vi "AcquisitionConfig.vi"(0 "frequency settings":T1={"frequency (Hz)"=0.001, "number of samples per cycle"=2.0, "number of cycles"=1.0} {"frequency (Hz)" min=0.001 max=100000000.0; "number of samples per cycle" min=2.0 step=1.0; "number of cycles" min=1.0}, 5 "channel settings":T2={"units"=10348, "input terminal configuration"=-1, "maximum value"=5.0, "minimum value"=-5.0} {"units" items=["Volts"=10348, "From Custom Scale"=10065]; "input terminal configuration" items=["Default"=-1, "RSE"=10083, "NRSE"=10078, "Differential"=10106, "Pseudodifferential"=12529]}, 7 "physical channels":tag, 11 "error in":errorcluster) -> (4 "task out":refnum<k21>, 8 "number of samples":dbl, 15 "error out":errorcluster)   [LabVIEW 2025]
uses:
  <vilib>/DAQmx/create/channels.llb/DAQmx Create Channel (AI-Voltage-Basic).vi
  <vilib>/DAQmx/configure/timing.llb/DAQmx Timing (Use Waveform).vi
panel:
  # "Configuración de la DAQ para\nadquisición de datos."
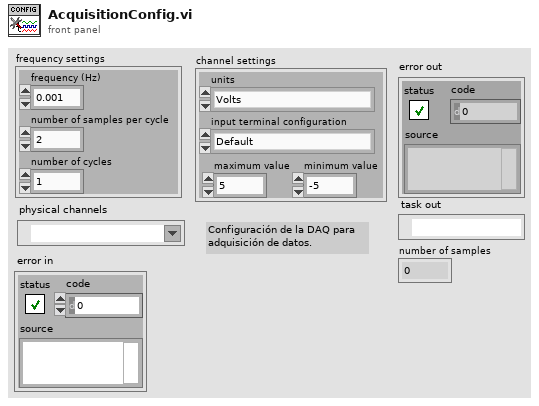
[diagram p1: front panel]
types:
  T1 = cluster{"frequency (Hz)":dbl, "number of samples per cycle":dbl, "number of cycles":dbl}
  T2 = cluster{"units":i32, "input terminal configuration":i32, "maximum value":dbl, "minimum value":dbl}
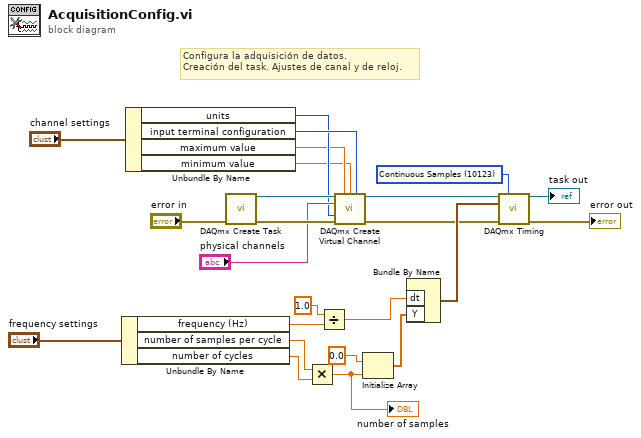
[diagram p0: block diagram]
diagram:
  w11 = 10123 items=["Finite Samples"=10178, "Continuous Samples"=10123, "Hardware Timed Single Point"=12522] ("sample mode")
  # "Configura la adquisición de datos.\nCreación del task. Ajustes de canal y de reloj."
  n1 = Unbundle By Name("frequency settings") -> ("frequency (Hz)"=w17:dbl, "number of samples per cycle"=w16:dbl, "number of cycles"=w15:dbl)
  n2 = Unbundle By Name("channel settings") -> ("units"=w4:i32, "input terminal configuration"=w5:i32, "maximum value"=w3:dbl, "minimum value"=w2:dbl)
  n3 = call <vilib>:"DAQmx Create Task.vi"("error in"="error in") -> ("task out"=w22:refnum<k21>, "error out"=w23:errorcluster)  [unwired: 13 in]
  n4 = Multiply(x=w16, y=w15) -> (x*y=w1:dbl)
  "number of samples" <- w1
  n5 = Divide(x=1.0, y=w17) -> (x/y=w20:dbl)
  n6 = call-poly <vilib>:"DAQmx Create Virtual Channel.vi"("task in"=w22, "maximum value"=w3, "minimum value"=w2, "input terminal configuration"=w5, "physical channels"="physical channels", "units"=w4, "error in"=w23) -> ("task out"=w10:refnum<k21>, "error out"=w9:errorcluster)  [unwired: 7 in]
  n7 = Initialize Array(0.0 ("element"), w1) -> (w13:dbl[])
  n8 = Bundle By Name("dt"=w20, "Y"=w13) -> (w12:waveform(dbl))  [unwired: 1 in]
  n9 = call-poly <vilib>:"DAQmx Timing.vi"("task/channels in"=w10, "sample mode"=w11, "waveform"=w12, "error in"=w9) -> ("task out"=→"task out":refnum<k21>, "error out"=→"error out":errorcluster)  [unwired: 10 in]
